vi "login.vi"(8 "error in":errorcluster, 11 "Device In":T1) -> (0 "error out":errorcluster, 3 "Device Out":T1)   [LabVIEW 2019]
uses:
  <userlib>/Onshape/_SubVI/Cluster.ctl
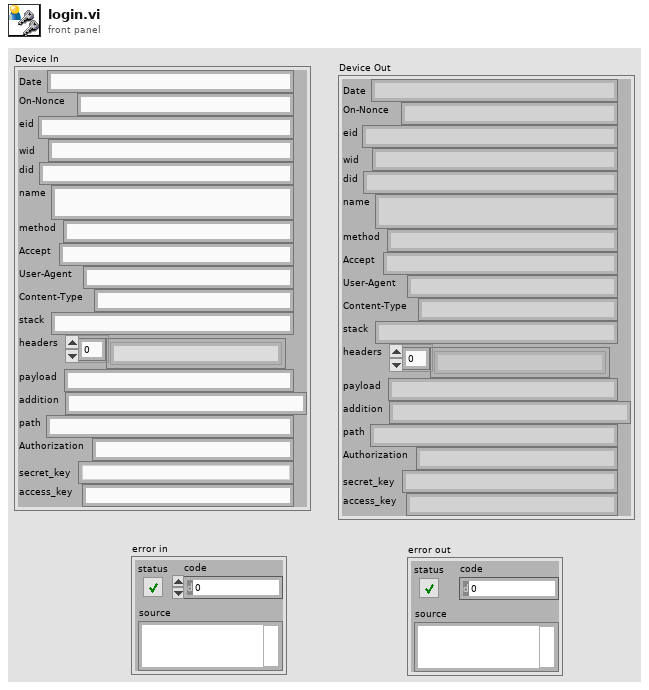
[diagram p1: front panel]
types:
  T1 = typedef "Cluster.ctl" = cluster{"Date":string, "On-Nonce":string, "eid":string, "wid":string, "did":string, "name":string, "method":string, "Accept":string, "User-Agent":string, "Content-Type":string, "stack":string, "headers":string[], "payload":string, "addition":string, "path":string, "Authorization":string, "secret_key":string, "access_key":string}
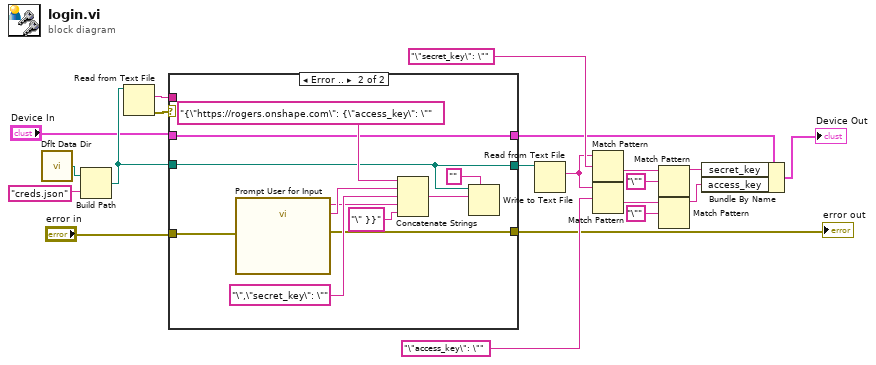
[diagram p0: block diagram]
diagram:
  n1 = call <vilib>:"Dflt Data Dir.vi"() -> ("App:Default Data Directory"=w8:path)
  n2 = Build Path(base path=w8, name or relative path="creds.json") -> (appended path=w6:path)
  n3 = Read from Text File(file (use dialog)=w6) -> (text=w19:string, error out=w20:errorcluster)  [unwired: 3 in, 2 out]
  n4 = case shown="Error .." w20 {
    tunnel: "Device In" -> [w22 w27]
    tunnel: w19 -> [_ _]
    tunnel: w6 -> [w21 w25]
    tunnel: [w22 w27] -> w10
    tunnel: [w21 w25] -> w5
    tunnel: "error in" -> [_ w24]
    tunnel: [_ w23] -> w1
    frame No Error {
    }
    frame Error {
      n5 = call "Prompt User for Input"("error in (no error)"=w24) -> ("secret_key"=w30:string, "access_key"=w32:string, "error out"=w23:errorcluster)  [unwired: 15 in, 1 out]
      n6 = Concatenate Strings("{\"https://rogers.onshape.com\": {\"access_key\": \"", w32, "\",\"secret_key\": \"", w30, "\" }}") -> (w28:string)
      n7 = Write to Text File(prompt (Choose or enter file path)="", file (use dialog)=w25, text=w28) -> ()  [unwired: 1 in, 3 out]
    }
  }
  "error out" <- w1
  n8 = Read from Text File(file (use dialog)=w5) -> (text=w9:string)  [unwired: 3 in, 3 out]
  n9 = Match Pattern(string=w9, regular expression="\"secret_key\": \"") -> (after substring=w15:string)  [unwired: 1 in, 3 out]
  n10 = Match Pattern(string=w9, regular expression="\"access_key\": \"") -> (after substring=w16:string)  [unwired: 1 in, 3 out]
  n11 = Match Pattern(string=w15, regular expression="\"") -> (before substring=w17:string)  [unwired: 1 in, 3 out]
  n12 = Match Pattern(string=w16, regular expression="\"") -> (before substring=w18:string)  [unwired: 1 in, 3 out]
  n13 = Bundle By Name(cluster=w10, "secret_key"=w17, "access_key"=w18) -> (→"Device Out":T1)
